vi "Sample (SubVI).vi"(11 "Temperature (F)":dbl) -> (3 "Numeric":dbl)   [LabVIEW 2024]
panel:
  in  "Boolean":bool
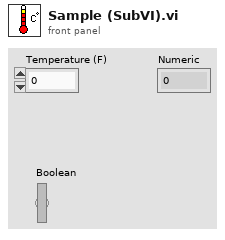
[diagram p1: front panel]
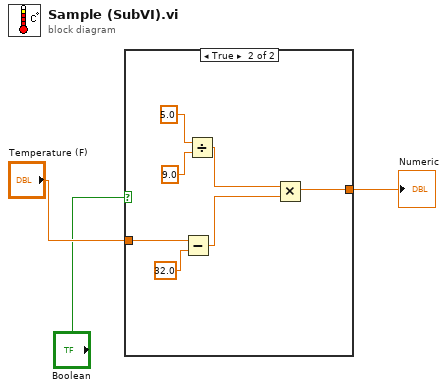
[diagram p0: block diagram]
diagram:
  n1 = case shown="True" "Boolean" {
    tunnel: "Temperature (F)" -> [w4 w10]
    tunnel: [w4 w9] -> w2
    frame False {
    }
    frame True {
      n2 = Subtract(x=w10, y=32.0) -> (x-y=w8:dbl)
      n3 = Divide(x=5.0, y=9.0) -> (x/y=w7:dbl)
      n4 = Multiply(x=w7, y=w8) -> (x*y=w9:dbl)
    }
  }
  "Numeric" <- w2
